vi "Set Default Control Style.vi"(8 "error in (no error)":errorcluster, 11 "vi path":path) -> (0 "error out":errorcluster)   [LabVIEW 2024]
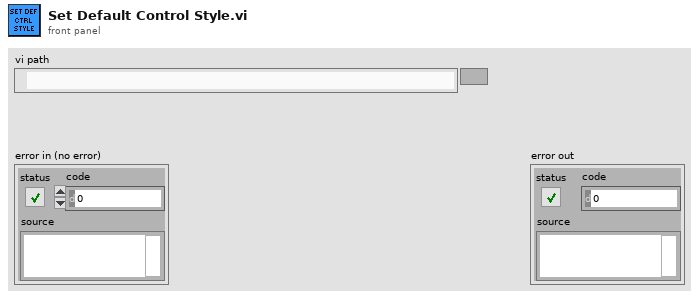
[diagram p1: front panel]
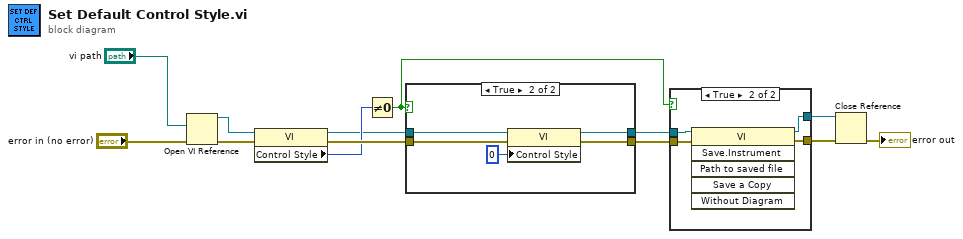
[diagram p0: block diagram]
diagram:
  n1 = Open VI Reference(vi path="vi path", error in (no error)="error in (no error)") -> (vi reference=w7:refnum<vi>, error out=w8:errorcluster)  [unwired: 4 in]
  n2 = property class="VI"(reference=w7, error in=w8) -> (reference out=w4:refnum<vi>, error out=w6:errorcluster, "Control Style"=w5:i32)
  n3 = Not Equal To 0?(x=w5) -> (x != 0?=w2:bool)
  n4 = case shown="True" w2 {
    tunnel: w6 -> [w15 w19]
    tunnel: [w15 w18] -> w1
    tunnel: w4 -> [w14 w17]
    tunnel: [w14 w16] -> w3
    frame False {
    }
    frame True {
      n5 = property class="VI"(reference=w17, error in=w19, "Control Style"=0) -> (reference out=w16:refnum<vi>, error out=w18:errorcluster)
    }
  }
  n6 = case shown="True" w2 {
    tunnel: [w22 w26] -> w10
    tunnel: [w21 w25] -> w9
    tunnel: w1 -> [w22 w24]
    tunnel: w3 -> [w21 w23]
    frame False {
    }
    frame True {
      n7 = invoke class="VI" method="Save.Instrument"(reference=w23, error in=w24) -> (reference out=w25:refnum<vi>, error out=w26:errorcluster)  [unwired: 4 in, 4 out]
    }
  }
  n8 = Close Reference(reference=w9, error in (no error)=w10) -> (error out=→"error out":errorcluster)
